vi "Delete Cycle.vi"(8 "Error In (no error)":errorcluster, 10 "Cycle":T1, 11 "SQLite DB Operator In":refnum<class "SQLite DB Operator.lvclass">) -> (0 "Error Out":errorcluster, 3 "SQLite DB Operator Out":refnum<class "SQLite DB Operator.lvclass">)   [LabVIEW 2023, in "SQLite DB Operator.lvclass"]
uses:
  SQLite DB Operator.lvclass
  SQLite DB Operator.lvclass/SQLite DB Operator.ctl
  DB Operator/Public/Ctrls/DB Controls/Cycle.ctl
  DB Operator/DB Operator.lvclass
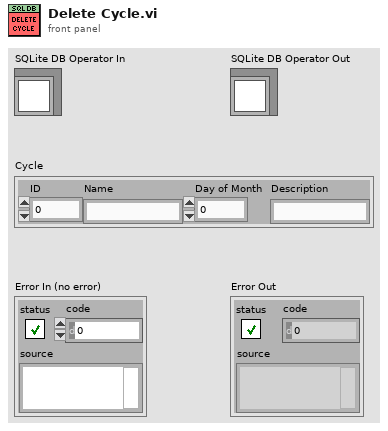
[diagram p1: front panel]
types:
  T1 = typedef "DB Operator.lvclass/Cycle.ctl" = cluster{"ID":u32, "Name":string, "Day of Month":u8, "Description":string}
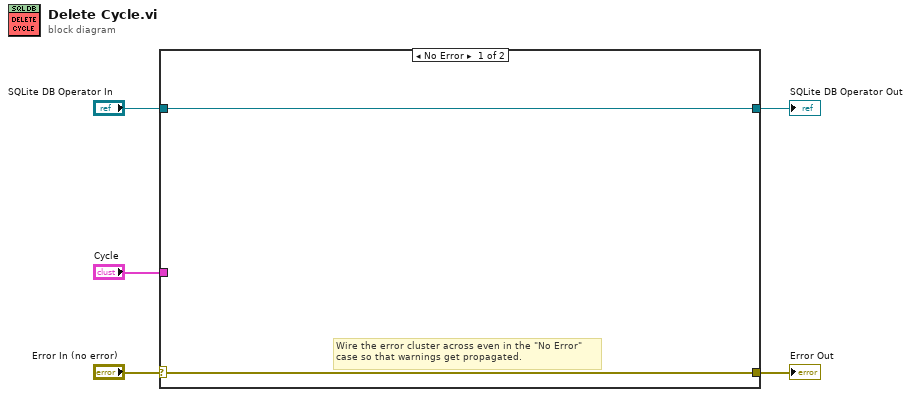
[diagram p0: block diagram]
diagram:
  n1 = case shown="No Error" "Error In (no error)" {
    selector: "Error In (no error)" -> [w6 w9]
    tunnel: [w6 w9] -> w3
    tunnel: [w7 w8] -> w4
    tunnel: "SQLite DB Operator In" -> [w7 w8]
    tunnel: "Cycle" -> [_ _]
    frame No Error {
      # "Wire the error cluster across even in the \"No Error\"\ncase so that warnings get propagated."
    }
    frame Error {
    }
  }
  "Error Out" <- w3
  "SQLite DB Operator Out" <- w4
